vi "AI Reg UI.vi"(8 "error in (no error)":errorcluster, 11 "Node Ptr":T2 format="%.0x") -> (0 "error out":errorcluster)   [LabVIEW 2021, in "Modbus Master System Explorer.lvlib"]
uses:
  Modbus Master System Explorer.lvlib
  <vilib>/NI VeriStand/Custom Device API/Custom Device Item Ref.ctl
  Shared/Controls/Data Model/DataType.ctl
  SubVIs/Modbus Type.ctl
  <vilib>/NI VeriStand/Custom Device API/Custom Device API.lvlib
  Shared/Modbus Master Shared.lvlib
panel:
  in  "Unit ID":u8
  out "Registers":i32
  in  "DataType":T1
  in  "Sub-Index (Bool)":u16
  in  "Valid?":string
  in  "Address":u16
  in  "Header":cluster{"Section Name":string}={"Section Name"="Input Register (Analog Input) Settings"}
  in  "Description":string
  in  "Name":string
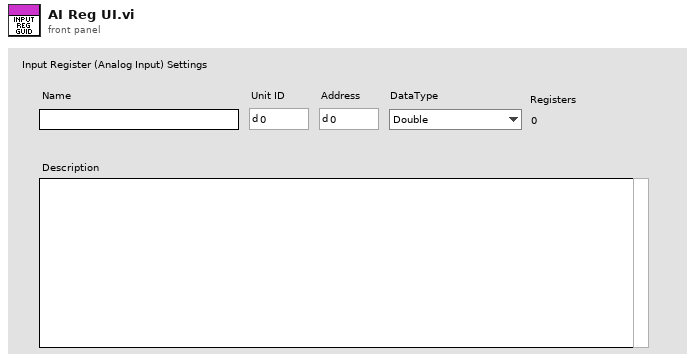
[diagram p1: front panel]
types:
  T1 = typedef "Modbus Master Shared.lvlib/DataType.ctl" = enum16{"Double", "Single", "I64", "I32", "I16", "I8", "U64", "U32", "U16", "U8", "Boolean"}
  T2 = typedef "Custom Device API.lvlib/Custom Device Item Ref.ctl" = u64
  T3 = typedef "Modbus Master Shared.lvlib/Modbus Type.ctl" = enum16{"Coil", "Discrete Input", "Holding Register", "Input Register"}
  T4 = typedef "Custom Device API.lvlib/Custom Device Commands.ctl" = enum16{"Default", "Item renamed", "Shutdown", "Dynamic button pressed"}
  T5 = typedef "Custom Device API.lvlib/Custom Device Item Info.ctl" = cluster{"Name":string, "Is Channel":bool, "GUID":string, "Is Waveform":bool}
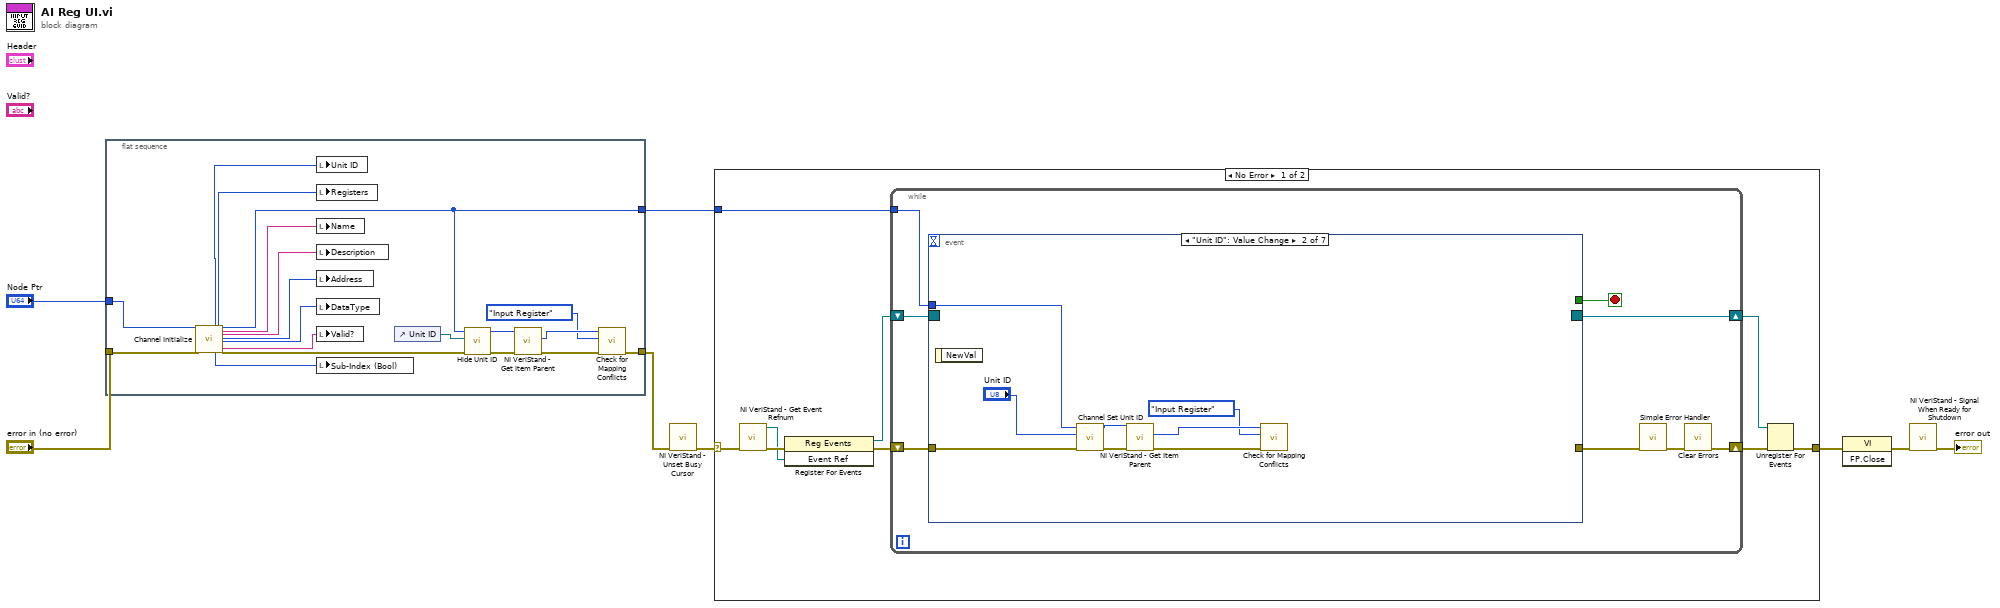
[diagram p0: block diagram]
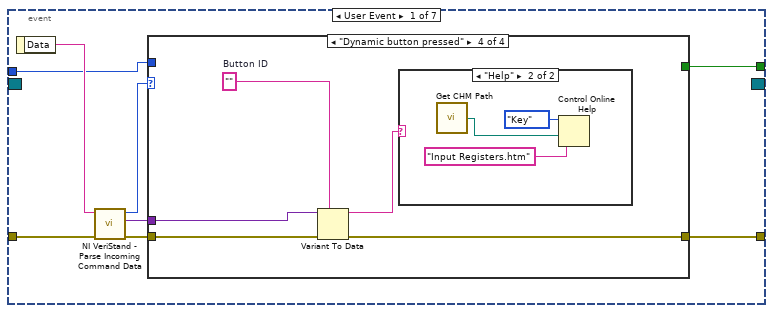
[diagram p2: hidden frame]
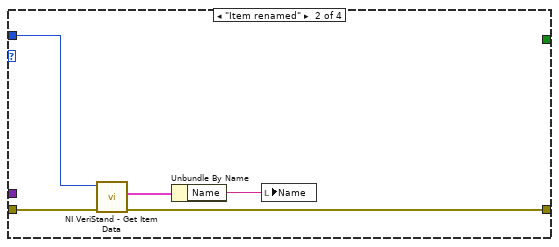
[diagram p4: hidden frame]
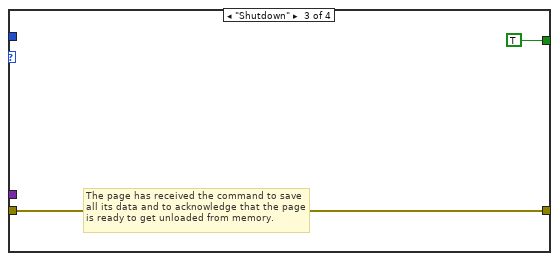
[diagram p5: hidden frame]
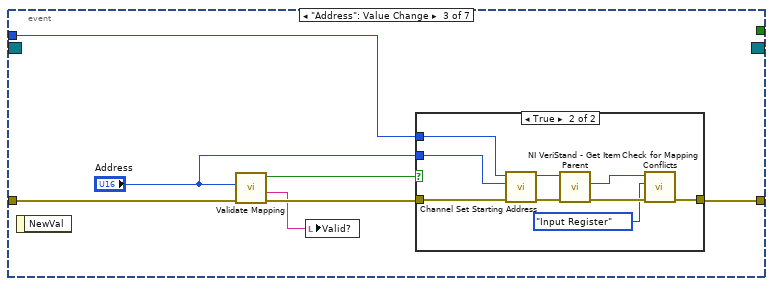
[diagram p7: hidden frame]
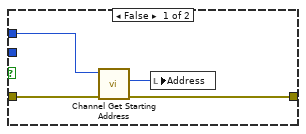
[diagram p8: hidden frame]
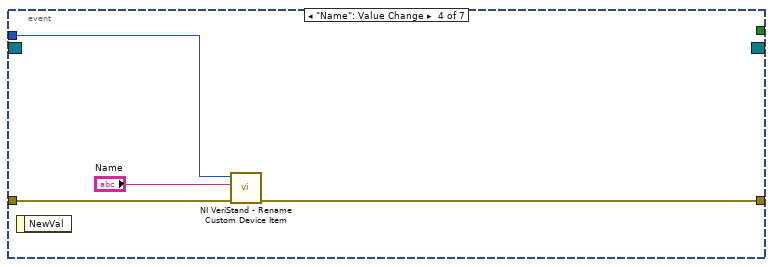
[diagram p9: hidden frame]
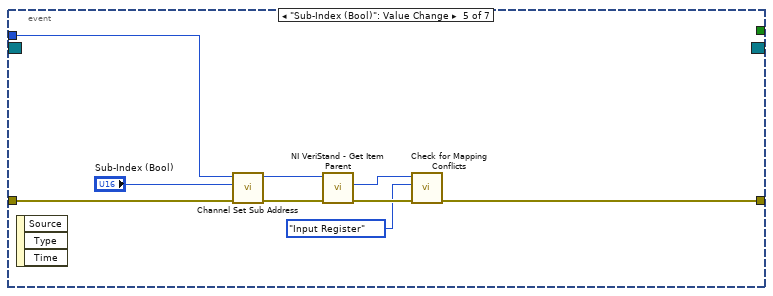
[diagram p10: hidden frame]
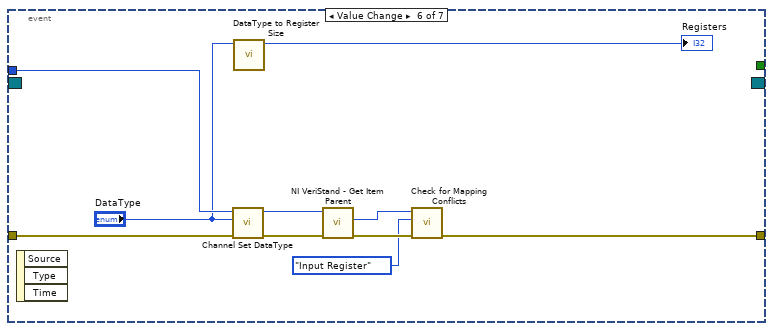
[diagram p11: hidden frame]
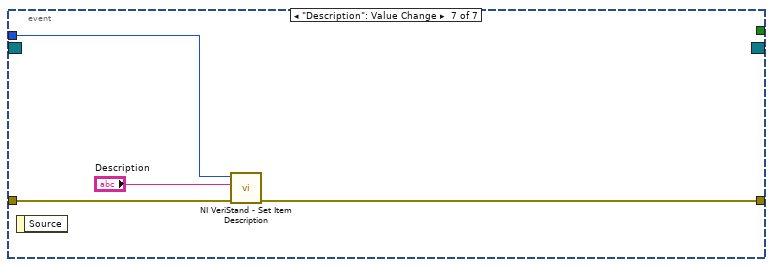
[diagram p12: hidden frame]
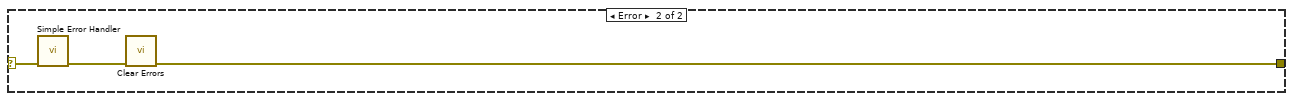
[diagram p13: hidden frame]
diagram:
  n1 = flat-sequence {
    tunnel: "Node Ptr" -> [w20]
    tunnel: [w11] -> w3
    tunnel: "error in (no error)" -> [w19]
    tunnel: [w14] -> w1
    frame #0 {
      n2 = call "Channel Initialize.vi"("Item Ref in"=w20, "error in (no error)"=w19) -> ("Unit ID"=w18:u8, "Sub-Index (Bool)"=w22:u16, "Registers"=w23:i32, "Channel Ref out"=w11:T2, "Name"=w26:string, "Description"=w27:string, "Starting Address"=w24:u16, "DataType"=w25:T1, "Status Message"=w21:string, "error out"=w10:errorcluster)  [unwired: 13 in, 3 out]
      n3 = local write "Unit ID"(w18) -> ()
      n4 = local write "Registers"(w23) -> ()
      n5 = local write "Name"(w26) -> ()
      n6 = local write "Description"(w27) -> ()
      n7 = local write "Address"(w24) -> ()
      n8 = local write "DataType"(w25) -> ()
      n9 = local write "Valid?"(w21) -> ()
      n10 = local write "Sub-Index (Bool)"(w22) -> ()
      n11 = control-ref of="Unit ID"() -> (w9:refnum<vi>)
      n12 = call "Hide Unit ID.vi"("error in (no error)"=w10, "Ctrl Ref"=w9, "Item Ref in"=w11) -> ("error out"=w13:errorcluster, "Item Ref out"=w12:T2)  [unwired: 7 in]
      n13 = call <vilib>:"NI VeriStand - Get Item Parent.vi"("error in (no error)"=w13, "Item Ref in"=w12) -> ("error out"=w15:errorcluster, "Parent Ref"=w17:T2)  [unwired: 6 in, 2 out]
      n14 = call "Check for Mapping Conflicts.vi"("error in (no error)"=w15, "Type"=Modbus_Type."Input Register", "Coiil Group Ref in in"=w17) -> ("error out"=w14:errorcluster)  [unwired: 5 in, 3 out]
    }
  }
  n15 = call <vilib>:"NI VeriStand - Unset Busy Cursor.vi"("error in (no error)"=w1) -> ("error out"=w5:errorcluster)  [unwired: 10 out]
  n16 = case shown="No Error" w5 {
    selector: w5 -> [w28 w126]
    tunnel: [w33 w124] -> w8
    tunnel: w3 -> [w29 _]
    frame No Error {
      n17 = call <vilib>:"NI VeriStand - Get Event Refnum.vi"("error in (no error)"=w28) -> ("error out"=w36:errorcluster, "Event Ref"=w32:refnum<user-event>)  [unwired: 9 out]
      n18 = register-events(error in=w36, w32) -> (reference out=w30:refnum<event-registration>, error out=w31:errorcluster)  [unwired: 1 in]
      n19 = while {
        tunnel: w29 -> [w40]
        shift-right: [w37] -> w34
        shift-left: w31 -> [w43]
        shift-right: [w44] -> w35
        shift-left: w30 -> [w42]
        stop <- w41 stop-if-true
        n20 = event shown="[1] \"Unit ID\": Value Change" {
          selector: w42 -> [_ _ _ _ _ _ _]
          dyn-events: [_ _ _ _ _ _ _] -> w44
          timeout: _ -> [_ _ _ _ _ _ _]
          tunnel: w43 -> [w52 w74 w81 w100 w107 w118 w122]
          tunnel: [w48 _ _ _ _ _ _] -> w41
          tunnel: [w47 _ w82 w99 w103 w113 w121] -> w39
          tunnel: w40 -> [w46 w76 w83 w98 w108 w119 w123]
          event User Event {
            n21 = event-data() -> ("Data"=w51:string)  [unwired: 1 out]
            n22 = call <vilib>:"NI VeriStand - Parse Incoming Command Data.vi"("error in (no error)"=w52, "Incoming data"=w51) -> ("error out"=w50:errorcluster, "Outgoing data"=w45:variant, "Action"=w49:T4)  [unwired: 7 out]
            n23 = case shown="\"Dynamic button pressed\"" w49 {
              tunnel: w50 -> [w53 w58 w59 w65]
              tunnel: [_ _ TRUE _] -> w48
              tunnel: [w53 w55 w59 w62] -> w47
              tunnel: w46 -> [_ w57 _ _]
              tunnel: w45 -> [_ _ _ w64]
              frame "Default", Default {
              }
              frame "Item renamed" {
                n24 = call <vilib>:"NI VeriStand - Get Item Data.vi"("error in (no error)"=w58, "Item Ref in"=w57) -> ("error out"=w55:errorcluster, "Item Info"=w56:T5)  [unwired: 8 out]
                n25 = Unbundle By Name(w56) -> ("Name"=w54:string)
                n26 = local write "Name"(w54) -> ()
              }
              frame "Shutdown" {
                # "The page has received the command to save all its data and to acknowledge that the page is ready to get unloaded from memory."
              }
              frame "Dynamic button pressed" {
                w63 = ""  # Button ID
                n27 = Variant To Data(error in=w65, type=w63, Variant=w64) -> (data=w61:string, error out=w62:errorcluster)
                n28 = case shown="\"Help\"" w61 {
                  frame Default {
                  }
                  frame "Help" {
                    n29 = call "Get CHM Path.vi"() -> ("appended path"=w68:path)
                    n30 = Control Online Help(2:w68, 3:"Input Registers.htm" ("String to search for"), 4:enum16{"Contents", "Key", "Close"}."Key" ("Operation")) -> ()  [unwired: 1 in, 1 out]
                  }
                }
              }
            }
          }
          event "Unit ID": Value Change {
            n31 = event-data() -> ()  [unwired: 2 out]
            n32 = call "Channel Set Unit ID.vi"("error in (no error)"=w74, "Value"="Unit ID", "Item Ref in"=w76) -> ("error out"=w69:errorcluster, "Item Ref out"=w70:T2)  [unwired: 7 in]
            n33 = call <vilib>:"NI VeriStand - Get Item Parent.vi"("error in (no error)"=w69, "Item Ref in"=w70) -> ("error out"=w72:errorcluster, "Parent Ref"=w73:T2)  [unwired: 6 in, 2 out]
            n34 = call "Check for Mapping Conflicts.vi"("error in (no error)"=w72, "Type"=Modbus_Type."Input Register", "Coiil Group Ref in in"=w73) -> ()  [unwired: 5 in, 4 out]
          }
          event "Address": Value Change {
            n35 = event-data() -> ()  [unwired: 2 out]
            n36 = call "Validate Mapping.vi"("error in (no error)"=w81, "Mapping"="Address") -> ("error out"=w80:errorcluster, "Status Message"=w79:string, "Valid?"=w78:bool)  [unwired: 7 in]
            n37 = local write "Valid?"(w79) -> ()
            n38 = case shown="True" w78 {
              tunnel: w83 -> [w87 w95]
              tunnel: [w84 w90] -> w82
              tunnel: w80 -> [w85 w96]
              tunnel: "Address" -> [_ w94]
              frame False {
                n39 = call "Channel Get Starting Address.vi"("error in (no error)"=w85, "Item Ref in"=w87) -> ("error out"=w84:errorcluster, "Value"=w86:u16)  [unwired: 7 in, 1 out]
                n40 = local write "Address"(w86) -> ()
              }
              frame True {
                n41 = call "Channel Set Starting Address.vi"("error in (no error)"=w96, "Value"=w94, "Item Ref in"=w95) -> ("error out"=w93:errorcluster, "Item Ref out"=w92:T2)  [unwired: 7 in]
                n42 = call <vilib>:"NI VeriStand - Get Item Parent.vi"("error in (no error)"=w93, "Item Ref in"=w92) -> ("error out"=w91:errorcluster, "Parent Ref"=w89:T2)  [unwired: 6 in, 2 out]
                n43 = call "Check for Mapping Conflicts.vi"("error in (no error)"=w91, "Type"=Modbus_Type."Input Register", "Coiil Group Ref in in"=w89) -> ("error out"=w90:errorcluster)  [unwired: 5 in, 3 out]
              }
            }
          }
          event "Name": Value Change {
            n44 = event-data() -> ()  [unwired: 2 out]
            n45 = call <vilib>:"NI VeriStand - Rename Custom Device Item.vi"("error in (no error)"=w100, "New Name"="Name", "Item Ref in"=w98) -> ("error out"=w99:errorcluster)  [unwired: 1 in, 7 out]
          }
          event "Sub-Index (Bool)": Value Change {
            n46 = event-data() -> ()  [unwired: 4 out]
            n47 = call "Channel Set Sub Address.vi"("error in (no error)"=w107, "Value"="Sub-Index (Bool)", "Item Ref in"=w108) -> ("error out"=w104:errorcluster, "Item Ref out"=w102:T2)  [unwired: 7 in]
            n48 = call <vilib>:"NI VeriStand - Get Item Parent.vi"("error in (no error)"=w104, "Item Ref in"=w102) -> ("error out"=w105:errorcluster, "Parent Ref"=w106:T2)  [unwired: 6 in, 2 out]
            n49 = call "Check for Mapping Conflicts.vi"("error in (no error)"=w105, "Type"=Modbus_Type."Input Register", "Coiil Group Ref in in"=w106) -> ("error out"=w103:errorcluster)  [unwired: 5 in, 3 out]
          }
          event Value Change {
            n50 = event-data() -> ()  [unwired: 4 out]
            n51 = call "Channel Set DataType.vi"("error in (no error)"=w118, "DataType"="DataType", "Item Ref in"=w119) -> ("error out"=w115:errorcluster, "Item Ref out"=w117:T2)  [unwired: 7 in]
            n52 = call "DataType to Register Size.vi"("DataType"="DataType") -> ("Registers"=→"Registers":i32)  [unwired: 9 in, 1 out]
            n53 = call <vilib>:"NI VeriStand - Get Item Parent.vi"("error in (no error)"=w115, "Item Ref in"=w117) -> ("error out"=w114:errorcluster, "Parent Ref"=w116:T2)  [unwired: 6 in, 2 out]
            n54 = call "Check for Mapping Conflicts.vi"("error in (no error)"=w114, "Type"=Modbus_Type."Input Register", "Coiil Group Ref in in"=w116) -> ("error out"=w113:errorcluster)  [unwired: 5 in, 3 out]
          }
          event "Description": Value Change {
            n55 = event-data() -> ()  [unwired: 2 out]
            n56 = call <vilib>:"NI VeriStand - Set Item Description.vi"("error in (no error)"=w122, "Description"="Description", "Item Ref in"=w123) -> ("error out"=w121:errorcluster)  [unwired: 8 out]
          }
        }
        n57 = call <vilib>:"Simple Error Handler.vi"("error in (no error)"=w39) -> ("error out"=w38:errorcluster)  [unwired: 1 in, 7 out]
        n58 = call <vilib>:"Clear Errors.vi"("error in (no error)"=w38) -> ("error out"=w37:errorcluster)  [unwired: 1 in, 5 out]
      }
      n59 = Unregister For Events(event registration refnum=w35, error in=w34) -> (error out=w33:errorcluster)
    }
    frame Error {
      n60 = call <vilib>:"Simple Error Handler.vi"("error in (no error)"=w126) -> ("error out"=w125:errorcluster)  [unwired: 1 in, 7 out]
      n61 = call <vilib>:"Clear Errors.vi"("error in (no error)"=w125) -> ("error out"=w124:errorcluster)  [unwired: 1 in, 5 out]
    }
  }
  n62 = invoke class="VI" method="FP.Close"(error in=w8) -> (error out=w7:errorcluster)  [unwired: 2 in, 2 out]
  n63 = call <vilib>:"NI VeriStand - Signal When Ready for Shutdown.vi"("error in (no error)"=w7) -> ("error out"=→"error out":errorcluster)  [unwired: 10 out]
